vi "ConsoleOut.vi"() -> ()   [LabVIEW 2017]
panel:
  in  "ConsoleOut":string
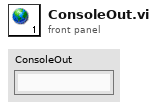
[diagram p1: front panel]
diagram:
